vi "SRS_QCM_simple.vi"(11 "SRS address in":T2={"SRS on?"=TRUE, "VISA in "="GPIB0::3::INSTR", "error in (no error)"={"status"=FALSE, "code"=0, "source"=""}}) -> (1 "Resistance out":dbl format="%.6f", 2 "Frequency out":dbl format="%.6f", 3 "SRS address out":T1)   [LabVIEW 2014]
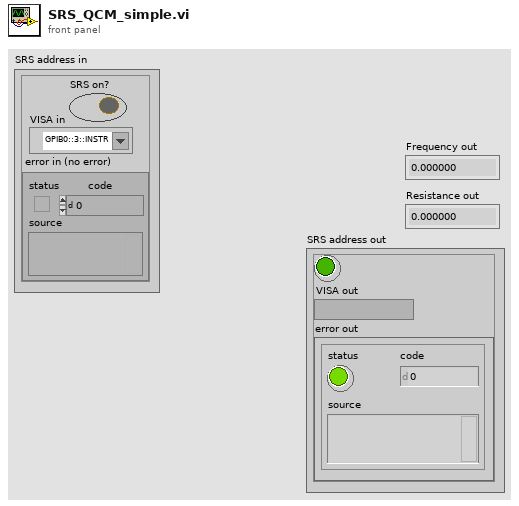
[diagram p1: front panel]
types:
  T1 = cluster{"Boolean":bool, "VISA out":refnum<visa-resource-name>, "error out":errorcluster}
  T2 = cluster{"SRS on?":bool, "VISA in ":refnum<visa-resource-name>, "error in (no error)":errorcluster}
  T3 = cluster{bool, "VISA out":refnum<visa-resource-name>, "error out":errorcluster}
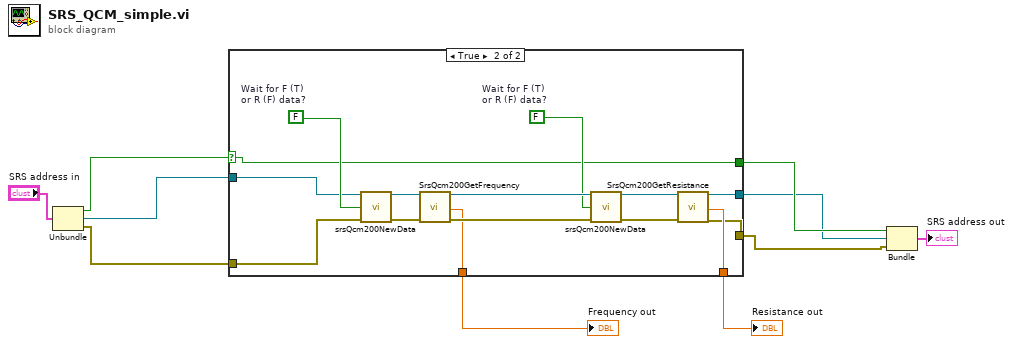
[diagram p0: block diagram]
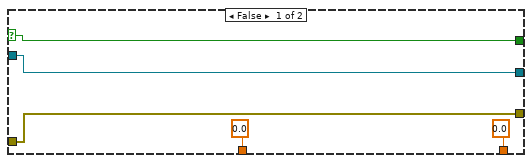
[diagram p2: hidden frame]
diagram:
  n1 = Unbundle("SRS address in") -> ("SRS on?"=w7:bool, "VISA in"=w6:refnum<visa-resource-name>, "error in (no error)"=w5:errorcluster)
  n2 = case shown="True" w7 {
    selector: w7 -> [w11 w16]
    tunnel: w6 -> [w13 w25]
    tunnel: w5 -> [w12 w24]
    tunnel: [w13 w22] -> w3
    tunnel: [0.0 ("Resistance out") w21] -> w10
    tunnel: [0.0 ("Frequency out") w18] -> w9
    tunnel: [w12 w17] -> w2
    tunnel: [w11 w16] -> w4
    frame False {
    }
    frame True {
      w27 = FALSE  # Wait for F (T) or R (F) data?
      w26 = FALSE  # Wait for F (T) or R (F) data?
      n3 = call "srsQcm200NewData.vi"("VISA in"=w25, "Wait for F (T)\nor R (F) data?"=w26, "error in (no error)"=w24) -> ("VISA out"=w30:refnum<visa-resource-name>, "error out"=w20:errorcluster)  [unwired: 11 in]
      n4 = call "SrsQcm200GetFrequency.vi"("VISA in"=w30, "error in (no error)"=w20) -> ("VISA out"=w28:refnum<visa-resource-name>, "Frequency out"=w18:dbl, "error out"=w29:errorcluster)  [unwired: 15 in]
      n5 = call "srsQcm200NewData.vi"("VISA in"=w28, "Wait for F (T)\nor R (F) data?"=w27, "error in (no error)"=w29) -> ("VISA out"=w23:refnum<visa-resource-name>, "error out"=w19:errorcluster)  [unwired: 11 in]
      n6 = call "SrsQcm200GetResistance.vi"("VISA in"=w23, "error in (no error)"=w19) -> ("VISA out"=w22:refnum<visa-resource-name>, "Resistance out"=w21:dbl, "error out"=w17:errorcluster)  [unwired: 15 in]
    }
  }
  "Frequency out" <- w9
  "Resistance out" <- w10
  n7 = Bundle(w4, "VISA out"=w3, "error out"=w2) -> (→"SRS address out":T3)  [unwired: 1 in]
